vi "To XML - Non-Aggregated - XML contains only test suite.vi"() -> ()   [LabVIEW 2013, in "JUnit XML Tests.lvlib" / "Test Suite.lvlib"]
uses:
  Test Suite.lvlib
  JUnit XML/Test Suite/Test Suite.lvclass/Test Suite.ctl
  JUnit XML/Test Suite/Test Suite.lvclass
  JUnit XML/Test Suite/Write Timestamp.vi
  <vilib>/xml/Close Reference(Node).vi
  <vilib>/addons/_JKI Toolkits/Caraya/classes/Assert/Assert Equal Value_Variant.vi
  <vilib>/addons/_JKI Toolkits/Caraya/classes/Test/Test.lvclass
  <vilib>/addons/_JKI Toolkits/Caraya/classes/Assert/Assert.lvclass
  <resource>/objmgr/DOMUserDefRef.rc
  <vilib>/xml/NI_XML.lvlib
panel:
  out "error out":errorcluster
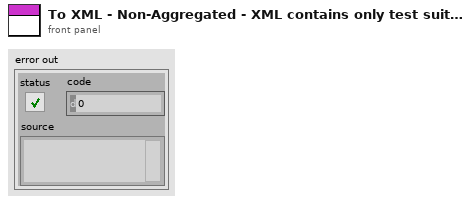
[diagram p1: front panel]
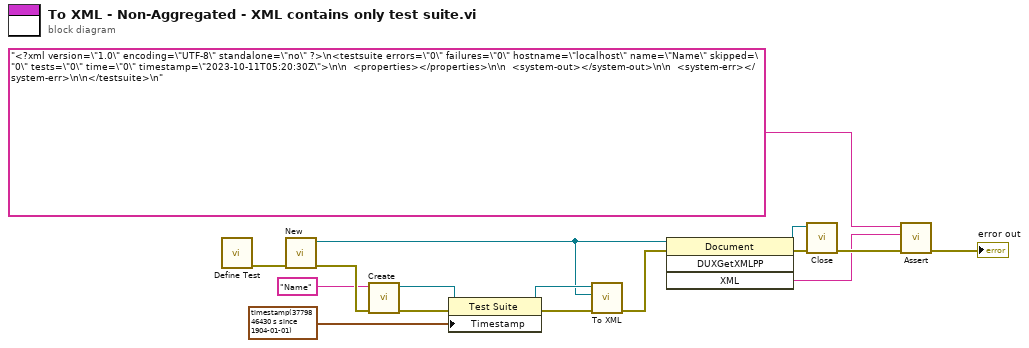
[diagram p0: block diagram]
diagram:
  n1 = call <vilib>:"Define Test.vi"() -> ("error out"=w16:errorcluster)  [unwired: 10 in, 1 out]
  n2 = call <vilib>:"New.vi"("error in (no error)"=w16) -> ("error out"=w14:errorcluster, "DOM document out"=w2:refnum<k20>)  [unwired: 7 in]
  n3 = call "Create.vi"("error in (no error)"=w14, "Name"="Name" ("Package")) -> ("error out"=w15:errorcluster, "Test Suite"=w6:refnum<class "Test Suite.lvclass">)  [unwired: 8 in]
  n4 = property class="Test Suite"(reference=w6, error in=w15, "Timestamp"=timestamp(3779846430.123 s since 1904-01-01)) -> (reference out=w5:refnum<class "Test Suite.lvclass">, error out=w7:errorcluster)
  n5 = call-dynamic "To XML.vi"("error in (no error)"=w7, "Parent"=w2, "Test Suite in"=w5) -> ("error out"=w1:errorcluster)  [unwired: 8 in]
  n6 = invoke class="Document" method="DUXGetXMLPP"(reference=w2, error in=w1) -> (reference out=w12:refnum<k20>, error out=w13:errorcluster, "XML"=w10:string)  [unwired: 2 in, 1 out]
  n7 = call-poly <vilib>:"Close.vi"("error in (no error)"=w13, "node"=w12) -> ("error out"=w11:errorcluster)  [unwired: 7 in]
  n8 = call-poly <vilib>:"Assert.vi"("error in (no error)"=w11, "Actual"=w10, "Expected"="<?xml version=\"1.0\" encoding=\"UTF-8\" standalone=\"no\" ?>\n<testsuite errors=\"0\" failures=\"0\" hostname=\"localhost\" name=\"Name\" skipped=\"0\" tests=\"0\" time=\"0\" timestamp=\"2023-10-11T05:20:30Z\">\n\n  <properties></properties>\n\n  <system-out></system-out>\n\n  <system-err></system-err>\n\n</testsuite>\n") -> ("error out"=→"error out":errorcluster)  [unwired: 7 in, 1 out]
